vi "Init.vi"(8 "error in (no error)":errorcluster, 11 "DAQ View in":refnum<class "DAQ View.lvclass">) -> (0 "error out":errorcluster, 3 "DAQ View out":refnum<class "DAQ View.lvclass">)   [LabVIEW 2022 SP3, in "DAQ View.lvclass"]
uses:
  DAQ View.lvclass
  DAQ View.lvclass/DAQ View.ctl
  iView/base view/base view.lvclass
  DAQ API/DAQ API.lvclass
  data.ctl
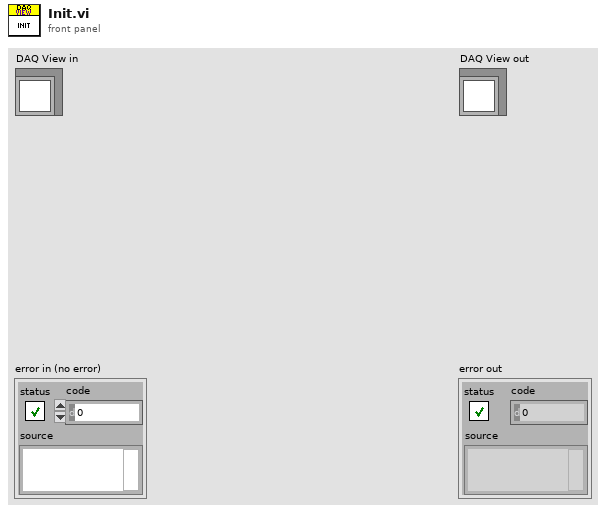
[diagram p1: front panel]
types:
  T1 = typedef "DAQ View.lvclass/data.ctl" = cluster{"DAQ API.lvclass":refnum<class "DAQ API.lvclass">}
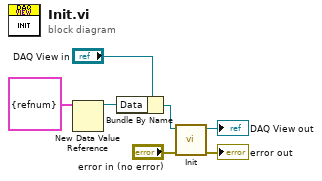
[diagram p0: block diagram]
diagram:
  n1 = New Data Value Reference(data value=T1 {"DAQ API.lvclass"=refnum} ("DATA")) -> (data value reference=w1:refnum<data-value>)  [unwired: 1 in, 1 out]
  n2 = Bundle By Name(cluster="DAQ View in", "Data"=w1) -> (w2:refnum<class "DAQ View.lvclass">)
  n3 = call-parent "Init.vi"("error in (no error)"="error in (no error)", "base view in"=w2) -> ("error out"=→"error out":errorcluster, "base view out"=→"DAQ View out":refnum<class "DAQ View.lvclass">)  [unwired: 8 in]
